vi "Unpack Script.vi"(1 "script":dbl[][](array[numeric]), 4 "index":i32) -> (13 "# of primitives":i32, 14 "primitive":i32, 15 "argument 1":dbl, 16 "argument 2":dbl, 17 "argument 3":dbl, 18 "argument 4":dbl, 19 "argument 5":dbl)   [LabVIEW 2014]
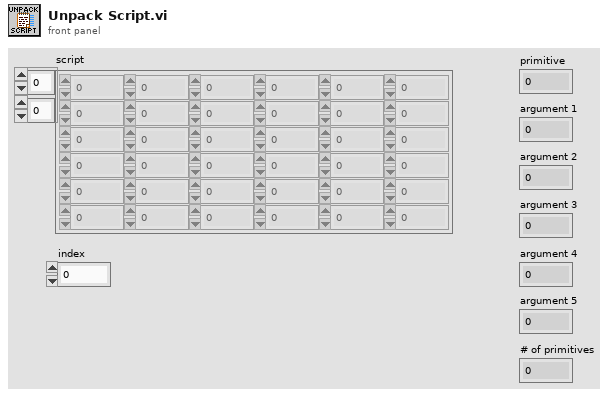
[diagram p1: front panel]
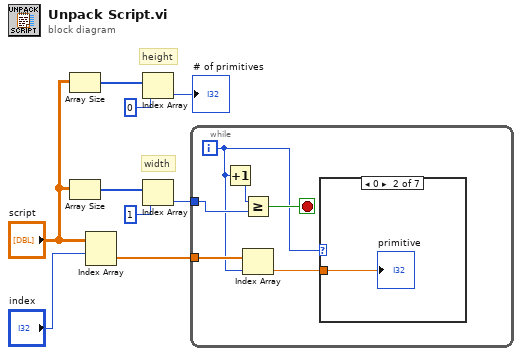
[diagram p0: block diagram]
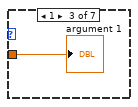
[diagram p3: hidden frame]
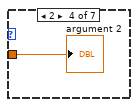
[diagram p4: hidden frame]
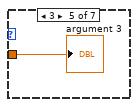
[diagram p5: hidden frame]
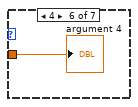
[diagram p6: hidden frame]
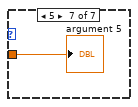
[diagram p7: hidden frame]
diagram:
  # "height"
  # "width"
  n1 = Array Size(array="script") -> (size(s)=w4:i32[])
  n2 = Array Size(array="script") -> (size(s)=w8:i32[])
  n3 = Index Array(array="script", index (row)="index") -> (element=w7:dbl[])  [unwired: 1 in]
  n4 = Index Array(array=w4, index=0) -> (element=→"# of primitives":i32)
  n5 = Index Array(array=w8, index=1) -> (element=w6:i32)
  n6 = while {
    tunnel: w7 -> [w15]
    tunnel: w6 -> [w12]
    i -> [w10]
    stop <- w11 stop-if-true
    n7 = Increment(x=w10) -> (x+1=w13:i32)
    n8 = Greater Or Equal?(x=w13, y=w12) -> (x >= y?=w11:bool)
    n9 = Index Array(array=w15, index=w10) -> (element=w14:dbl)
    n10 = case shown="0" w10 {
      tunnel: w14 -> [_ w16 w17 w18 w19 w20 w21]
      frame -1, Default {
      }
      frame 0 {
        "primitive" <- w16
      }
      frame 1 {
        "argument 1" <- w17
      }
      frame 2 {
        "argument 2" <- w18
      }
      frame 3 {
        "argument 3" <- w19
      }
      frame 4 {
        "argument 4" <- w20
      }
      frame 5 {
        "argument 5" <- w21
      }
    }
  }
